vi "Add FPGA Section.vi"(8 "error in (no error)":errorcluster, 9 "Channel Type":T3, 10 "User defined IOVs":T2(array[cluster]), 11 "Item Ref in":T1 format="%.0x") -> (0 "error out":errorcluster, 3 "Item Ref out":T1 format="%.0x")   [LabVIEW 2019, in "SEECD System Explorer.lvlib"]
uses:
  SEECD System Explorer.lvlib
  <vilib>/NI VeriStand/Custom Device API/Custom Device Channel Type.ctl
  <vilib>/NI VeriStand/Custom Device API/Custom Device Item Ref.ctl
  <vilib>/NI VeriStand/Custom Device API/Custom Device Channel.ctl
  Shared/Type Defs/FXP Config.ctl
  Shared/Globals/Scan Engine GUIDs.vi
  Shared/Globals/Property Strings.vi
  <vilib>/NI VeriStand/Custom Device API/Custom Device API.lvlib
  Shared/SEECD Shared.lvlib
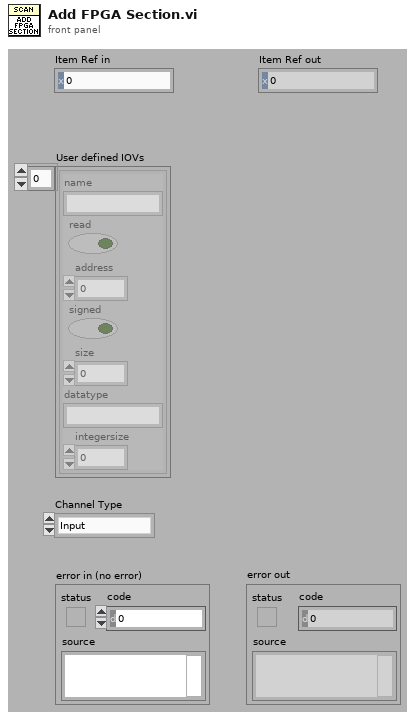
[diagram p1: front panel]
types:
  T1 = typedef "Custom Device API.lvlib/Custom Device Item Ref.ctl" = u64
  T2 = cluster{"name":string, "read":bool, "address":u32, "signed":bool, "size":u32, "datatype":string, "integersize":i32}[]
  T3 = typedef "Custom Device API.lvlib/Custom Device Channel Type.ctl" = enum16{"Input", "Output"}
  T4 = typedef "SEECD Shared.lvlib/FXP Config.ctl" = cluster{"signed":bool, "size":u32, "integersize":i32}
  T5 = typedef "Custom Device API.lvlib/Custom Device Channel.ctl" = cluster{"Type":T3, "Units":string, "Default Value":dbl, "Faultable":bool, "Scalable":bool}
  T6 = typedef "SEECD Shared.lvlib/UDV Data Type.ctl" = enum16{"Boolean", "Fixed Point", "Int8", "Int16", "Int32", "Int64", "U32 Bit Field", "UInt8", "UInt16", "UInt32", "UInt64", "Other", "DBL", "SGL"}
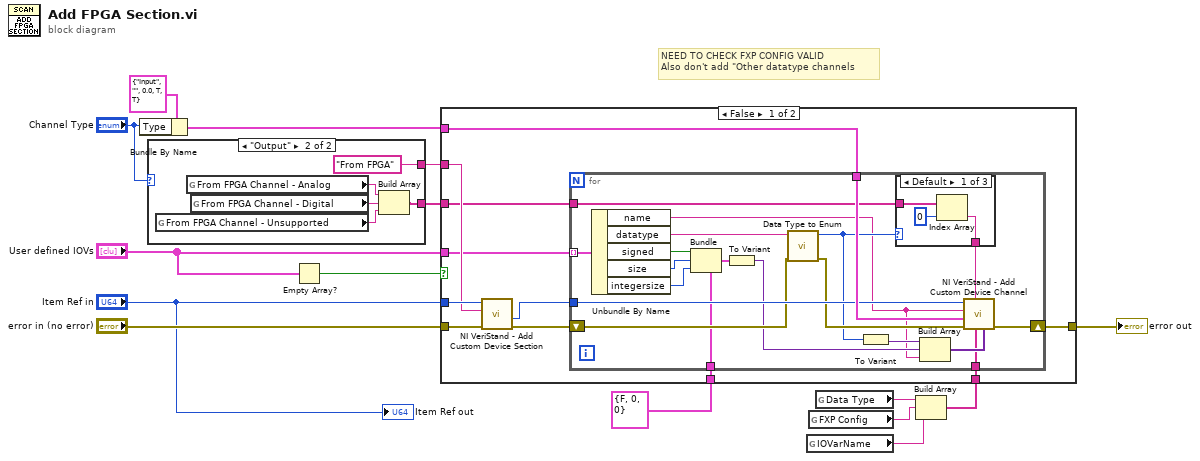
[diagram p0: block diagram]
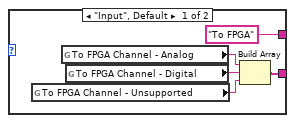
[diagram p2: hidden frame]
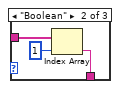
[diagram p3: hidden frame]
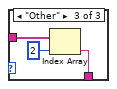
[diagram p4: hidden frame]
diagram:
  # "NEED TO CHECK FXP CONFIG VALID\nAlso don't add \"Other datatype channels"
  n1 = Bundle By Name(cluster=T5 {"Type"=enum."Input", "Units"="", "Default Value"=0.0, "Faultable"=TRUE, "Scalable"=TRUE} ("To 9144 Channel"), "Type"="Channel Type") -> (w10:T5)
  n2 = case shown="\"Output\"" "Channel Type" {
    tunnel: ["To FPGA" ("Section Name") "From FPGA" ("Section Name")] -> w9
    tunnel: [w16 w21] -> w3
    frame "Input", Default {
      n3 = global read "Scan Engine GUIDs.vi" "To FPGA Channel - Unsupported"() -> (w17:string)
      n4 = global read "Scan Engine GUIDs.vi" "To FPGA Channel - Analog"() -> (w19:string)
      n5 = global read "Scan Engine GUIDs.vi" "To FPGA Channel - Digital"() -> (w18:string)
      n6 = Build Array(w19, w18, w17) -> (w16:string[])
    }
    frame "Output" {
      n7 = global read "Scan Engine GUIDs.vi" "From FPGA Channel - Unsupported"() -> (w24:string)
      n8 = global read "Scan Engine GUIDs.vi" "From FPGA Channel - Analog"() -> (w22:string)
      n9 = global read "Scan Engine GUIDs.vi" "From FPGA Channel - Digital"() -> (w23:string)
      n10 = Build Array(w22, w23, w24) -> (w21:string[])
    }
  }
  n11 = Empty Array?(array="User defined IOVs") -> (empty?=w14:bool)
  n12 = global read "Property Strings.vi" "IOVarName"() -> (w1:string)
  n13 = global read "Property Strings.vi" "FXP Config"() -> (w5:string)
  n14 = global read "Property Strings.vi" "Data Type"() -> (w6:string)
  n15 = Build Array(w6, w5, w1) -> (w4:string[])
  n16 = case shown="False" w14 {
    tunnel: "error in (no error)" -> [w36 w66]
    tunnel: [w30 w66] -> w13
    tunnel: "Item Ref in" -> [w35 _]
    tunnel: w10 -> [w31 _]
    tunnel: w9 -> [w34 _]
    tunnel: "User defined IOVs" -> [w33 _]
    tunnel: w4 -> [w28 _]
    tunnel: w3 -> [w27 _]
    tunnel: T4 {"signed"=FALSE, "size"=0, "integersize"=0} ("FXP Config") -> [w26 _]
    frame False {
      n17 = call <vilib>:"NI VeriStand - Add Custom Device Section.vi"("error in (no error)"=w36, "Section Name"=w34, "Parent Ref in"=w35) -> ("error out"=w32:errorcluster, "Section Ptr"=w29:T1)  [unwired: 5 in, 2 out]
      n18 = for {
        tunnel: w33 -> [w53] mode=indexing
        shift-right: [w56] -> w30
        shift-left: w32 -> [w48]
        tunnel: w31 -> [w55]
        tunnel: w29 -> [w54]
        tunnel: w28 -> [w42]
        tunnel: w27 -> [w39]
        tunnel: w26 -> [w41]
        n19 = Unbundle By Name(w53) -> ("name"=w37:string, "datatype"=w49:string, "signed"=w52:bool, "size"=w51:u32, "integersize"=w50:i32)
        n20 = Bundle(cluster=w41, "signed"=w52, "size"=w51, "integersize"=w50) -> (w46:T4)
        n21 = To Variant(anything=w46) -> (Variant=w44:variant)
        n22 = call "Data Type to Enum.vi"("error in (no error)"=w48, "datatype in"=w49) -> ("error out"=w47:errorcluster, "UDV Data Type out"=w40:T6)  [unwired: 7 in]
        n23 = To Variant(anything=w40) -> (Variant=w45:variant)
        n24 = case shown="Default" w40 {
          tunnel: w39 -> [w58 w61 w64]
          tunnel: [w57 w60 w63] -> w38
          frame Default {
            n25 = Index Array(array=w58, index=0) -> (element=w57:string)
          }
          frame "Boolean" {
            n26 = Index Array(array=w61, index=1) -> (element=w60:string)
          }
          frame "Other" {
            n27 = Index Array(array=w64, index=2) -> (element=w63:string)
          }
        }
        n28 = Build Array(w45, w44, w37) -> (w43:variant[])
        n29 = call <vilib>:"NI VeriStand - Add Custom Device Channel.vi"("Property Values"=w43, "Property names"=w42, "GUID (Default Channel)"=w38, "error in (no error)"=w47, "Channel"=w55, "Channel Name"=w37, "Parent Ref in"=w54) -> ("error out"=w56:errorcluster)  [unwired: 1 in, 3 out]
      }
    }
    frame True {
    }
  }
  "error out" <- w13
  "Item Ref out" <- "Item Ref in"
